vi "ErrorToTemperature.vi"(3 "Input polarity?":bool, 4 "Rset":dbl=10000.0, 5 "Vref":dbl=1.0, 6 "Rgain":dbl=100000.0 format="%#_13g", 7 "PID reading":dbl format="%#_13g") -> (0 "Voltage / V":dbl, 1 "Temperature / C":dbl=25.0 format="%0.2f")   [LabVIEW 2014]
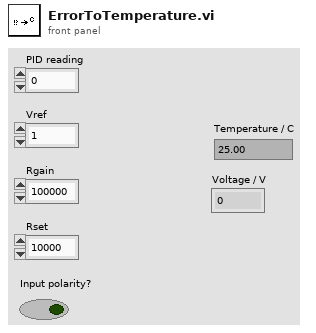
[diagram p1: front panel]
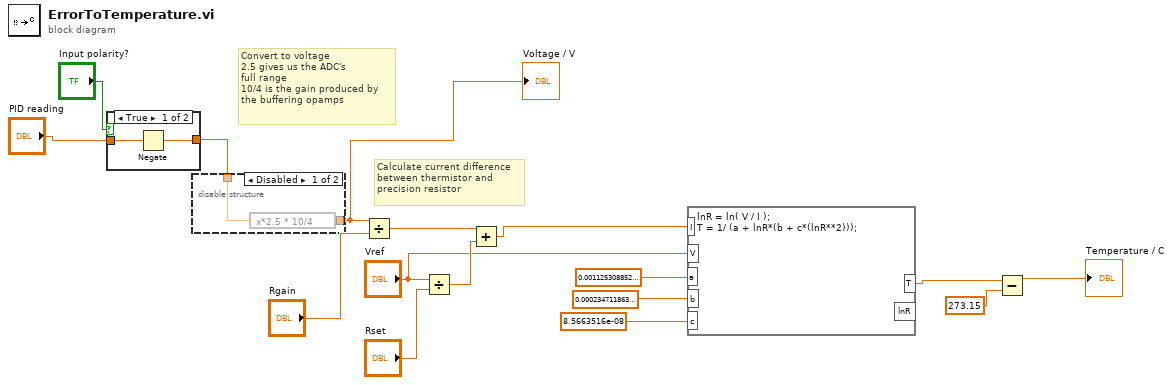
[diagram p0: block diagram]
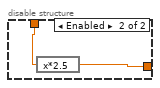
[diagram p3: hidden frame]
diagram:
  # "Calculate current difference\nbetween thermistor and\nprecision resistor"
  # "Convert to voltage\n2.5 gives us the ADC's \nfull range\n10/4 is the gain produced by \nthe buffering opamps"
  n1 = case shown="True" "Input polarity?" {
    tunnel: [w17 w19] -> w2
    tunnel: "PID reading" -> [w18 w19]
    frame True {
      n2 = Negate(x=w18) -> (-x=w17:dbl)
    }
    frame False {
    }
  }
  n3 = disable-structure shown="Disabled" {
    disable-tunnel: w2 -> [w21 w22]
    disable-tunnel: [w20 w23] -> w4
    frame Disabled {
      n4 = expression code="x*2.5 * 10/4"(w21) -> (w20:dbl)
    }
    frame Enabled {
      n5 = expression code="x*2.5"(w22) -> (w23:dbl)
    }
  }
  "Voltage / V" <- w4
  n6 = Divide(x=w4, y="Rgain") -> (x/y=w15:dbl)
  n7 = Divide(x="Vref", y="Rset") -> (x/y=w13:dbl)
  n8 = Add(x=w15, y=w13) -> (x+y=w11:dbl)
  n9 = formula code="lnR = ln( V / I );\nT = 1/ (a + lnR*(b + c*(lnR**2)));"("V"="Vref", "a"=0.001125308852122, "b"=0.000234711863267, "c"=8.5663516e-08, "I"=w11) -> ("T"=w10:dbl)  [unwired: 1 out]
  n10 = Subtract(x=w10, y=273.15) -> (x-y=→"Temperature / C":dbl)
